vi "BINI Input Clusters ArchiveAndFtp.vi"() -> (0 "Bini Error out":errorcluster, 3 "Bini Load":T1={"Site ID"="", "File Management cluster"={"Comp File Size"=FALSE, "File Handle Method"=enum."Archive and zip in place from file *.ext list", "file extention list"=[]}, "time stamp"=timestamp(0 s since 1904-01-01), "File output directories"={"Archive Location"=path "", "Archive Location 2"=path "<Not A Path>", "OutPut Path"=path "", "Directory(s) To Scan Files"=[]}, "Auto FTP"=FALSE, "Auto Archive"=FALSE, "FTP CRED Cluster"={"Host"="", "UserName"="", "PassWord"="", "FTP File Path"="", "Timeout (S)"=60, "ActivePasive"=FALSE, "Binary Ascii"=FALSE, "Remote Port"=21}, "hours old date mod(hours)"=2, "Email Notification Cluster"={"Mail Server"="", "Return Address"="", "Email User Name"="", "Password"=""}, "Email Recipiant List"=[], "Addresses to Ping"=[]} {"FTP CRED Cluster"."Timeout (S)" min=0 max=300 step=1})   [LabVIEW 2012]
uses:
  Bini ArchiveAndFtpCluster.ctl
  Controls/File Management.ctl
  Controls/File Path directories.ctl
  Controls/FTP Credintials.ctl
  Controls/Ping address and email notify.ctl
  Controls/PingElements.ctl
  <vilib>/Utility/sysdir.llb/System Directory Type.ctl
panel:
  # "File Handling Method"
  # "Passive"
  # "Active"
  # "Binary"
  # "Ascii"
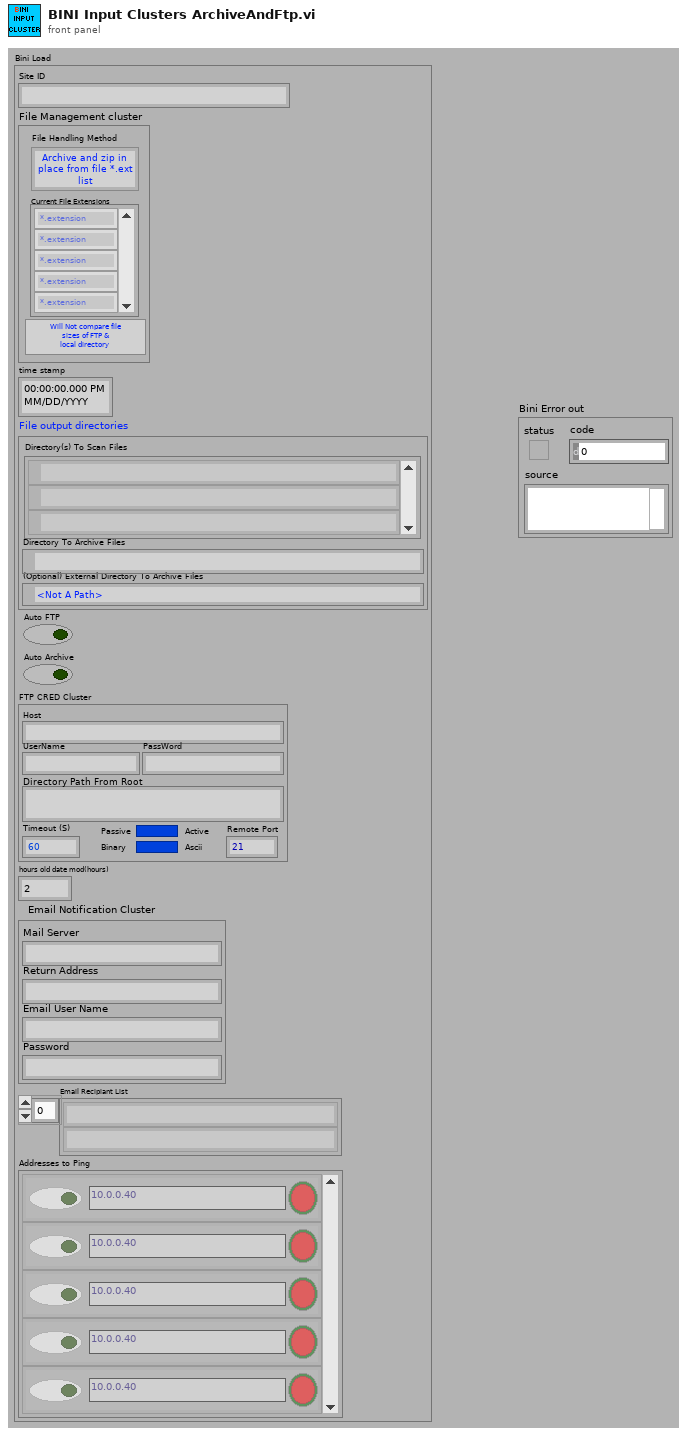
[diagram p1: front panel]
types:
  T1 = typedef "Bini ArchiveAndFtpCluster.ctl" = cluster{"Site ID":string, "File Management cluster":T2, "time stamp":timestamp, "File output directories":T3, "Auto FTP":bool, "Auto Archive":bool, "FTP CRED Cluster":T4, "hours old date mod(hours)":u8, "Email Notification Cluster":T5, "Email Recipiant List":string[], "Addresses to Ping":T6}
  T2 = typedef "File Management.ctl" = cluster{"Comp File Size":bool, "File Handle Method":enum16{"Archive and zip in place from file *.ext list", "Archive and zip ALL file Types to archive directory", "Archive and zip to archive directory from file *.ext list", "Perform no file management"}, "file extention list":string[]}
  T3 = typedef "File Path directories.ctl" = cluster{"Archive Location":path, "Archive Location 2":path, "OutPut Path":path, "Directory(s) To Scan Files":path[]}
  T4 = typedef "FTP Credintials.ctl" = cluster{"Host":string, "UserName":string, "PassWord":string, "FTP File Path":string, "Timeout (S)":i32, "ActivePasive":bool, "Binary Ascii":bool, "Remote Port":u16}
  T5 = typedef "Ping address and email notify.ctl" = cluster{"Mail Server":string, "Return Address":string, "Email User Name":string, "Password":string}
  T6 = typedef "PingElements.ctl" = cluster{"AddressNode 1":string, "Response 1":bool, "Ping on Address 1":bool}[]
  T7 = enum16{"open", "replace", "create", "open or create", "replace or create", "replace or create with confirmation"}
  T8 = typedef "System Directory Type.ctl" = i32
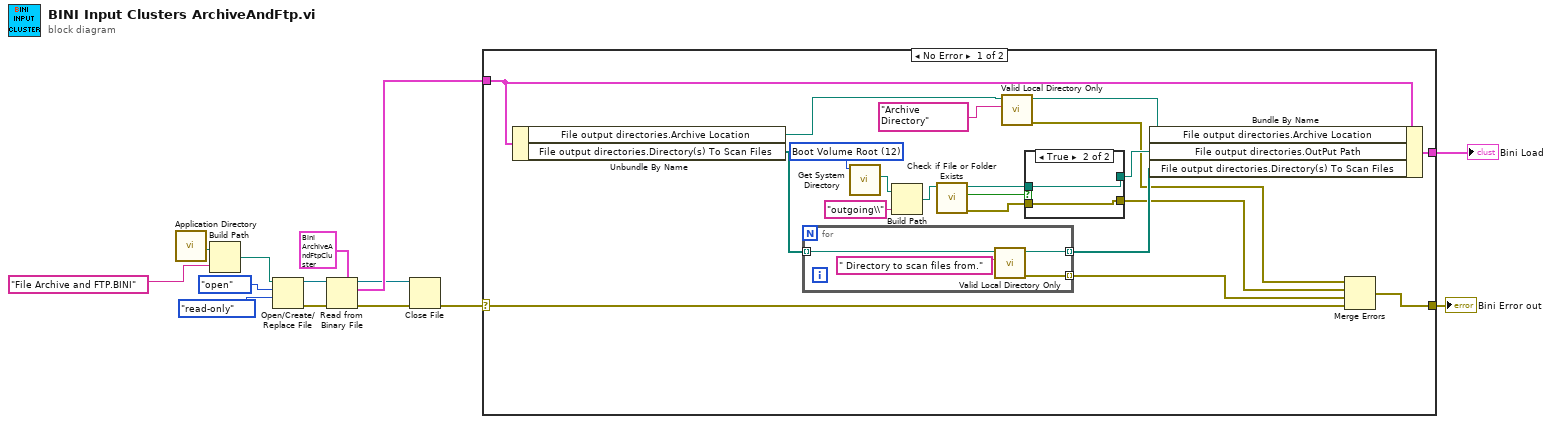
[diagram p0: block diagram]
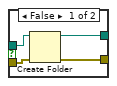
[diagram p2: hidden frame]
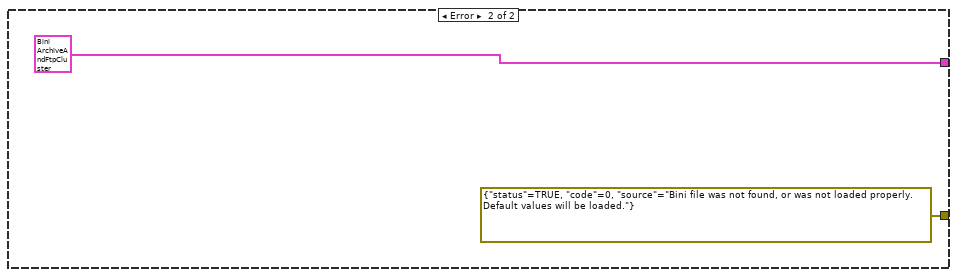
[diagram p3: hidden frame]
diagram:
  n1 = call <vilib>:"Application Directory.vi"() -> ("Application Directory"=w13:path)
  n2 = Build Path(base path=w13, name or relative path="File Archive and FTP.BINI") -> (appended path=w8:path)
  n3 = Open/Create/Replace File(file path (use dialog)=w8, operation (0:open)=T7."open", access (0:read/write)=enum16{"read/write", "read-only", "write-only"}."read-only") -> (refnum out=w9:refnum<file>, error out=w10:errorcluster)  [unwired: 3 in, 1 out]
  n4 = Read from Binary File(5:T1 {"Site ID"="", "File Management cluster"={"Comp File Size"=FALSE, "File Handle Method"=enum."Archive and zip in place from file *.ext list", "file extention list"=[]}, "time stamp"=timestamp(0 s since 1904-01-01), "File output directories"={"Archive Location"=path "", "Archive Location 2"=path "<Not A Path>", "OutPut Path"=path "", "Directory(s) To Scan Files"=[]}, "Auto FTP"=FALSE, "Auto Archive"=FALSE, "FTP CRED Cluster"={"Host"="", "UserName"="", "PassWord"="", "FTP File Path"="", "Timeout (S)"=60, "ActivePasive"=FALSE, "Binary Ascii"=FALSE, "Remote Port"=0}, "hours old date mod(hours)"=2, "Email Notification Cluster"={"Mail Server"="", "Return Address"="", "Email User Name"="", "Password"=""}, "Email Recipiant List"=[], "Addresses to Ping"=[]}, 8:w10, 11:w9) -> (0:w4:errorcluster, 2:w11:T1, 3:w5:refnum<file>)  [unwired: 3 in, 1 out]
  n5 = Close File(refnum=w5, error in=w4) -> (error out=w3:errorcluster)  [unwired: 1 out]
  n6 = case shown="No Error" w3 {
    selector: w3 -> [w34 _]
    tunnel: w11 -> [w33 _]
    tunnel: [w32 T1 {"Site ID"="", "File Management cluster"={"Comp File Size"=FALSE, "File Handle Method"=enum."Archive and zip in place from file *.ext list", "file extention list"=[]}, "time stamp"=timestamp(0 s since 1904-01-01), "File output directories"={"Archive Location"=path "", "Archive Location 2"=path "<Not A Path>", "OutPut Path"=path "", "Directory(s) To Scan Files"=[]}, "Auto FTP"=FALSE, "Auto Archive"=FALSE, "FTP CRED Cluster"={"Host"="", "UserName"="", "PassWord"="", "FTP File Path"="", "Timeout (S)"=60, "ActivePasive"=FALSE, "Binary Ascii"=FALSE, "Remote Port"=0}, "hours old date mod(hours)"=2, "Email Notification Cluster"={"Mail Server"="", "Return Address"="", "Email User Name"="", "Password"=""}, "Email Recipiant List"=[], "Addresses to Ping"=[]}] -> w2
    tunnel: [w19 errorcluster {"status"=TRUE, "code"=0, "source"="Bini file was not found, or was not loaded properly. Default values will be loaded."} ("error IO")] -> w1
    frame No Error {
      w28 = T8 12 items=["User Home"=0, "User Desktop"=1, "User Documents"=2, "User Application Data"=3, "User Preferences"=4, "User Temporary"=5, "Public Documents"=6, "Public Application Data"=7, "Public Preferences"=8, "Public Cache"=13, "System Core Libraries"=9, "System Installed Libraries"=10, "Application Files"=11, "Boot Volume Root"=12] ("system directory type")
      n7 = Unbundle By Name(w33) -> ("File output directories.Archive Location"=w23:path, "File output directories.Directory(s) To Scan Files"=w21:path[])
      n8 = for {
        tunnel: w21 -> [w37] mode=indexing
        tunnel: [w36] -> w20 mode=indexing
        tunnel: [w35] -> w17 mode=indexing
        n9 = call "Valid Local Directory Only.vi"("Directory ref"=" Directory to scan files from.", "Path input"=w37) -> ("error out"=w35:errorcluster, "Path output"=w36:path)  [unwired: 8 in]
      }
      n10 = call <vilib>:"Get System Directory.vi"("system directory type"=w28) -> ("system directory"=w29:path)  [unwired: 10 in]
      n11 = Build Path(base path=w29, name or relative path="outgoing\\") -> (appended path=w26:path)
      n12 = call <vilib>:"Check if File or Folder Exists.vi"("path"=w26) -> ("error out"=w18:errorcluster, "file or folder exists?"=w30:bool, "dup path"=w31:path)  [unwired: 8 in]
      n13 = call "Valid Local Directory Only.vi"("Directory ref"="Archive Directory", "Path input"=w23) -> ("error out"=w15:errorcluster, "Path output"=w22:path)  [unwired: 8 in]
      n14 = case shown="True" w30 {
        tunnel: w31 -> [w42 w44]
        tunnel: [w41 w44] -> w25
        tunnel: w18 -> [w40 w43]
        tunnel: [w39 w43] -> w16
        frame False {
          n15 = Create Folder(path (use dialog)=w42, error in=w40) -> (created path=w41:path, error out=w39:errorcluster)  [unwired: 1 in, 1 out]
        }
        frame True {
        }
      }
      n16 = Bundle By Name(cluster=w33, "File output directories.Archive Location"=w22, "File output directories.OutPut Path"=w25, "File output directories.Directory(s) To Scan Files"=w20) -> (w32:T1)
      n17 = Merge Errors(w15, w16, w17, w34) -> (w19:errorcluster)
    }
    frame Error {
    }
  }
  "Bini Load" <- w2
  "Bini Error out" <- w1
